vi "readSelectedGoal.vi"(8 "error in (no error)":errorcluster, 10 "WhichMonth.lvclass":refnum<class "WhichMonth.lvclass">, 11 "GoalUserInterface in":refnum<class "OutcomeListUIAdapter.lvclass">) -> (0 "error out":errorcluster, 2 "Goal.lvclass":refnum<class "Goal.lvclass">, 3 "GoalUserInterface out":refnum<class "OutcomeListUIAdapter.lvclass">)   [LabVIEW 2020, in "OutcomeListUIAdapter.lvclass"]
uses:
  OutcomeListUIAdapter.lvclass
  Goal/Goal.lvclass
  WhichMonth/WhichMonth.lvclass
  <vilib>/Utility/miscctls.llb/LVRowAndColumnTypeDef.ctl
  OutcomeListUIAdapter.lvclass/OutcomeListUIAdapter.ctl
  AbstractMultiColumnListBoxAdapter/AbstractMultiColumnListBoxAdapter.lvclass
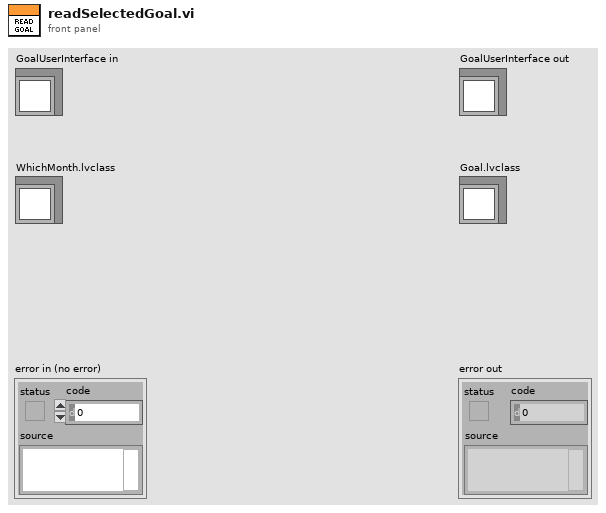
[diagram p1: front panel]
types:
  T1 = typedef "LVRowAndColumnTypeDef.ctl" = cluster{"Row":i32, "Column":i32}
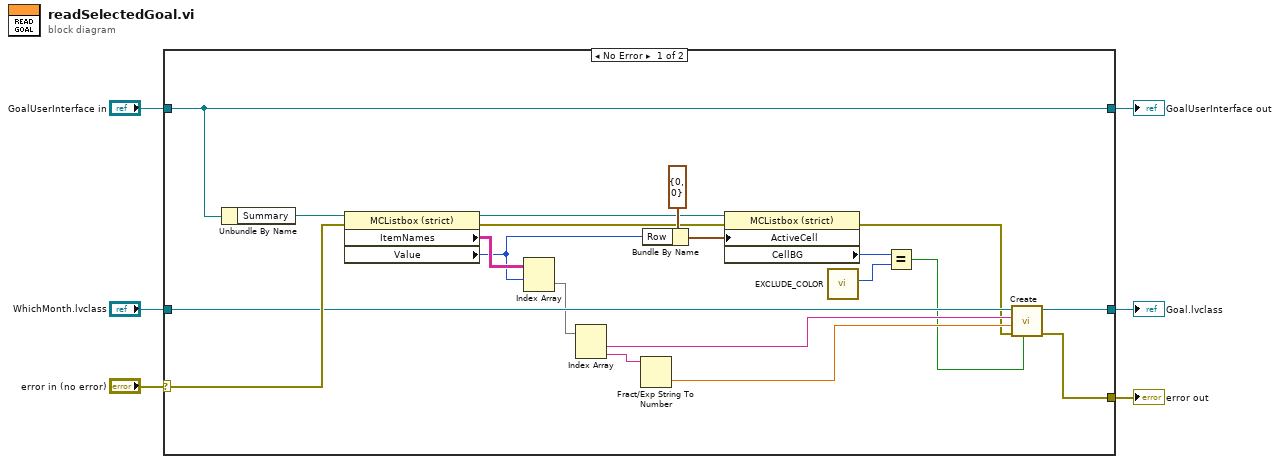
[diagram p0: block diagram]
diagram:
  n1 = case shown="No Error" "error in (no error)" {
    selector: "error in (no error)" -> [w25 w28]
    tunnel: [w23 w28] -> w5
    tunnel: [w11 w27] -> w3
    tunnel: "GoalUserInterface in" -> [w11 w27]
    tunnel: [w22 _] -> w2
    tunnel: "WhichMonth.lvclass" -> [w21 _]
    frame No Error {
      n2 = Unbundle By Name(w11) -> ("Summary"=w26:refnum<vi>)
      n3 = property class="MCListbox (strict)"(reference=w26, error in=w25) -> (reference out=w14:refnum<vi>, error out=w12:errorcluster, "ItemNames"=w24:string[][], "Value"=w13:i32)
      n4 = Index Array(array=w24, index (row)=w13) -> (element=w19:string[])  [unwired: 1 in]
      n5 = Index Array(array=w19) -> (element #1=w18:string, element #2=w17:string)  [unwired: 2 in]
      n6 = Fract/Exp String To Number(string=w17) -> (number=w20:dbl)  [unwired: 3 in, 1 out]
      n7 = Bundle By Name(cluster=T1 {"Row"=0, "Column"=0} ("Active Cell:Active Cell"), "Row"=w13) -> (w15:T1)
      n8 = property class="MCListbox (strict)"(reference=w14, error in=w12, "ActiveCell"=w15) -> (error out=w10:errorcluster, "CellBG"=w9:u32)  [unwired: 1 out]
      n9 = call "EXCLUDE_COLOR.vi"() -> ("Color Box"=w7:u32)  [unwired: 11 in]
      n10 = Equal?(x=w9, y=w7) -> (x = y?=w8:bool)
      n11 = call "Create.vi"("Exclude"=w8, "error in (no error)"=w10, "Amount"=w20, "Category Name"=w18, "WhichMonth.lvclass"=w21) -> ("error out"=w23:errorcluster, "Goal out"=w22:refnum<class "Goal.lvclass">)  [unwired: 5 in]
    }
    frame Error {
    }
  }
  "error out" <- w5
  "GoalUserInterface out" <- w3
  "Goal.lvclass" <- w2
